vi "Labview_360.vi"() -> ()   [LabVIEW 2020]
panel:
  out "Temperature":dbl(slide) scale=0.0..100.0
  in  "VISA resource name":refnum<visa-resource-name>
  out "Smoke Chart":dbl(graph)
  out "PIR Chart":dbl(graph)
  out "Smoke":dbl(slide) scale=0.0..1.0
  out "PIR":dbl(slide) scale=0.0..1.0
  out "Humidity":bool
  out "Fan":bool
  out "Light":bool
  out "Human Presence":bool
  out "Fire Indicator":bool
  in  "Table Control":string[][](table)
  out "Humidity":dbl(knob) scale=0.0..100.0
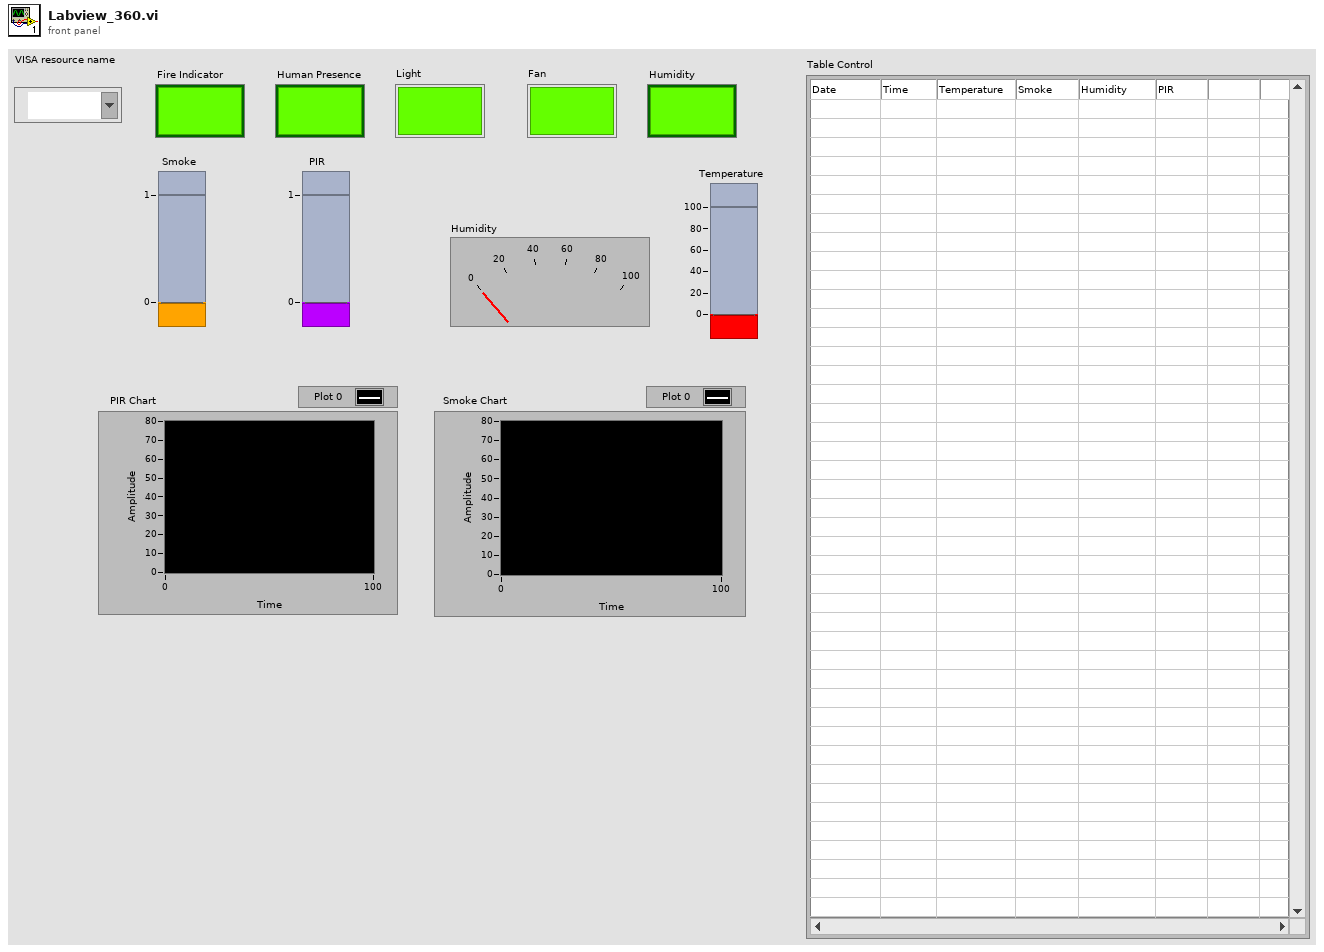
[diagram p1: front panel]
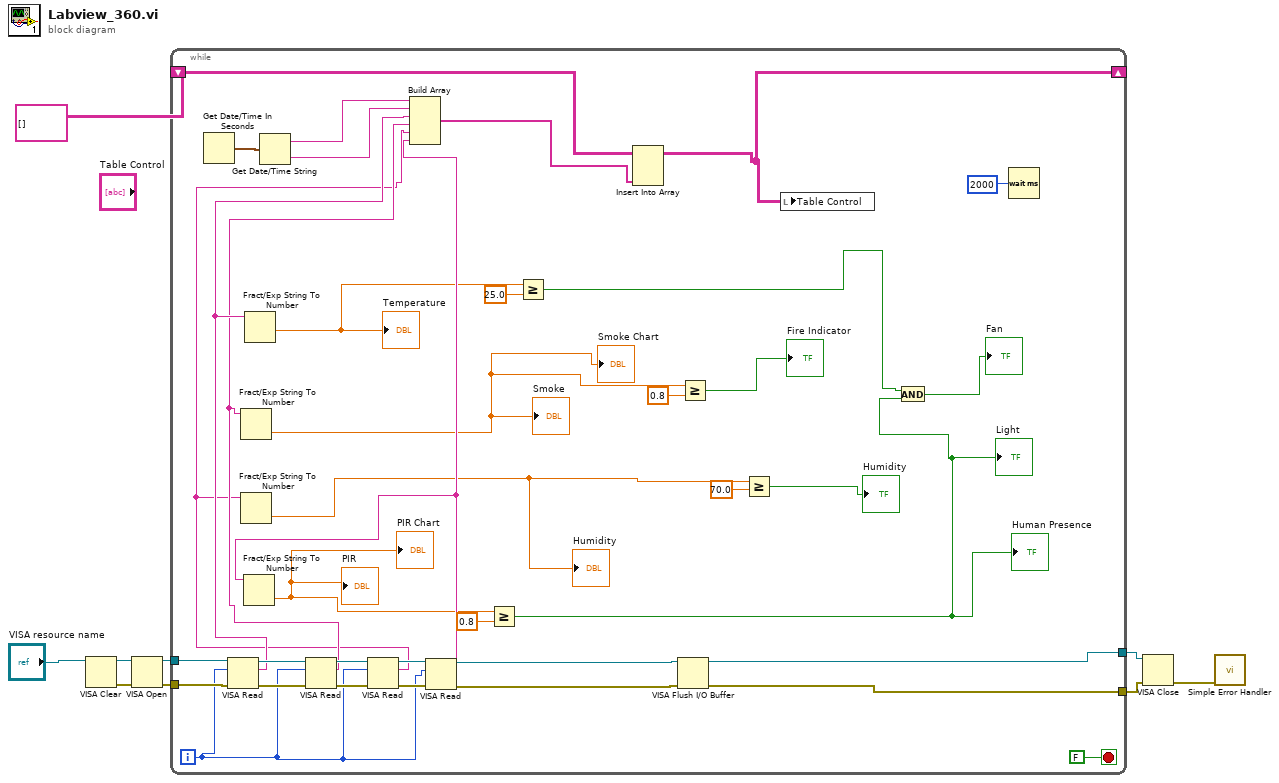
[diagram p0: block diagram]
diagram:
  n1 = VISA Clear(VISA resource name="VISA resource name") -> (VISA resource name out=w8:refnum<visa-resource-name>, error out=w9:errorcluster)  [unwired: 1 in]
  n2 = VISA Open(error in (no error)=w9, VISA resource name=w8) -> (VISA resource name=w7:refnum<visa-resource-name>, error out=w6:errorcluster)  [unwired: 3 in]
  n3 = while {
    tunnel: w7 -> [w41]
    tunnel: w6 -> [w40]
    tunnel: [w37] -> w5
    tunnel: [w36] -> w4
    shift-right: [w33] -> _
    shift-left: string[][] [] -> [w32]
    i -> [w35]
    stop <- FALSE stop-if-true
    n4 = Get Date/Time In Seconds() -> (seconds since 1Jan1904=w31:timestamp)
    n5 = VISA Read(VISA resource name=w41, byte count=w35, error in (no error)=w40) -> (VISA resource name out=w46:refnum<visa-resource-name>, read buffer=w26:string, error out=w47:errorcluster)  [unwired: 1 out]
    n6 = Fract/Exp String To Number(string=w26) -> (number=w22:dbl)  [unwired: 3 in, 1 out]
    "Temperature" <- w22
    n7 = Get Date/Time String(seconds (now)=w31) -> (date string=w30:string, time string=w29:string)  [unwired: 2 in]
    n8 = VISA Read(VISA resource name=w46, byte count=w35, error in (no error)=w47) -> (VISA resource name out=w44:refnum<visa-resource-name>, read buffer=w25:string, error out=w45:errorcluster)  [unwired: 1 out]
    n9 = Fract/Exp String To Number(string=w25) -> (number=w20:dbl)  [unwired: 3 in, 1 out]
    "Smoke" <- w20
    "Smoke Chart" <- w20
    n10 = VISA Read(VISA resource name=w44, byte count=w35, error in (no error)=w45) -> (VISA resource name out=w42:refnum<visa-resource-name>, read buffer=w23:string, error out=w43:errorcluster)  [unwired: 1 out]
    n11 = Fract/Exp String To Number(string=w23) -> (number=w10:dbl)  [unwired: 3 in, 1 out]
    "Humidity" <- w10
    n12 = VISA Read(VISA resource name=w42, byte count=w35, error in (no error)=w43) -> (VISA resource name out=w39:refnum<visa-resource-name>, read buffer=w24:string, error out=w38:errorcluster)  [unwired: 1 out]
    n13 = Fract/Exp String To Number(string=w24) -> (number=w15:dbl)  [unwired: 3 in, 1 out]
    "PIR" <- w15
    "PIR Chart" <- w15
    n14 = Build Array(w30, w29, w26, w25, w23, w24) -> (w28:string[])
    n15 = Greater Or Equal?(x=w15, y=0.8) -> (x >= y?=w13:bool)
    "Human Presence" <- w13
    "Light" <- w13
    n16 = Greater Or Equal?(x=w22, y=25.0) -> (x >= y?=w12:bool)
    n17 = Insert Into Array(array=w32, new element=w28) -> (w33:string[][])  [unwired: 2 in]
    n18 = VISA Flush I/O Buffer(VISA resource name=w39, error in (no error)=w38) -> (VISA resource name out=w37:refnum<visa-resource-name>, error out=w36:errorcluster)  [unwired: 1 in]
    n19 = Greater Or Equal?(x=w20, y=0.8) -> (x >= y?=→"Fire Indicator":bool)
    n20 = Greater Or Equal?(x=w10, y=70.0) -> (x >= y?=→"Humidity":bool)
    n21 = local write "Table Control"(w33) -> ()
    n22 = And(x=w12, y=w13) -> (x .and. y?=→"Fan":bool)
    n23 = Wait (ms)(milliseconds to wait=u32 2000) -> ()  [unwired: 1 out]
  }
  n24 = VISA Close(VISA resource name=w5, error in (no error)=w4) -> (error out=w3:errorcluster)
  n25 = call <vilib>:"Simple Error Handler.vi"("error in (no error)"=w3) -> ()  [unwired: 4 in, 5 out]
